vi "main.vi"() -> ()   [LabVIEW 2016]
panel:
  out "Y":dbl(slide) scale=0.0..720.0
  out "X":dbl(slide) scale=0.0..1280.0
  out "Ball Y Position":dbl
  out "Ball X Position":dbl
  out "Frame Rate":dbl
  in  "Stop (F)":bool
  out "Image Out":T1(plugin-control)
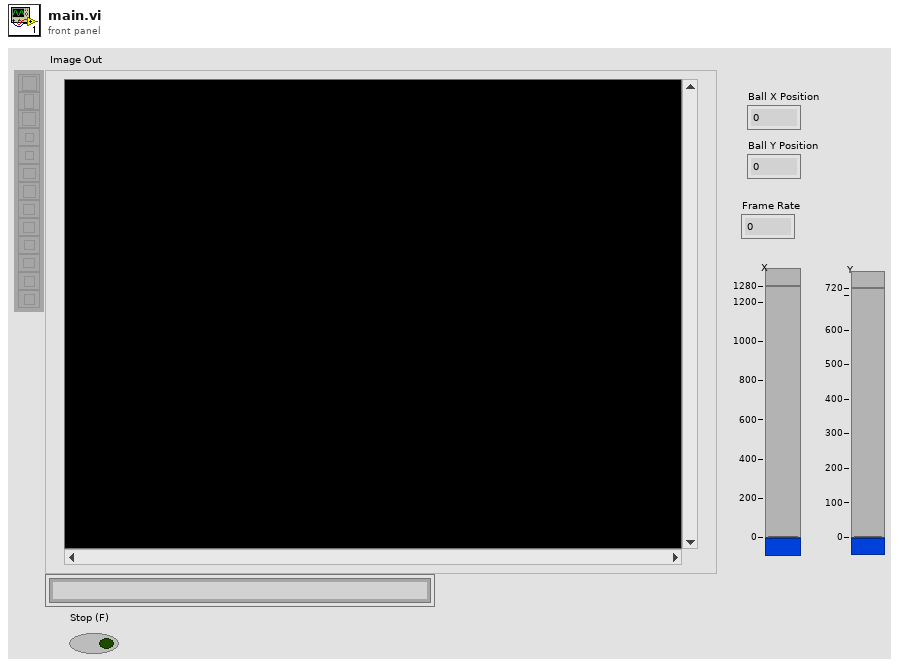
[diagram p1: front panel]
types:
  T1 = typedef "IMAQ Image.ctl" = refnum<image>
  T2 = cluster{"Label":string, "Score":i32, "Angle":dbl, "Location":cluster{"X":dbl, "Y":dbl}, "Bounding Box":cluster{"X":dbl, "Y":dbl}[], "Object Found?":bool}[]
  T3 = cluster{"Label":string, "Score":i32, "Angle":dbl, "Location":cluster{"X":dbl, "Y":dbl}, "Bounding Box":cluster{"X":dbl, "Y":dbl}[], "Object Found?":bool}
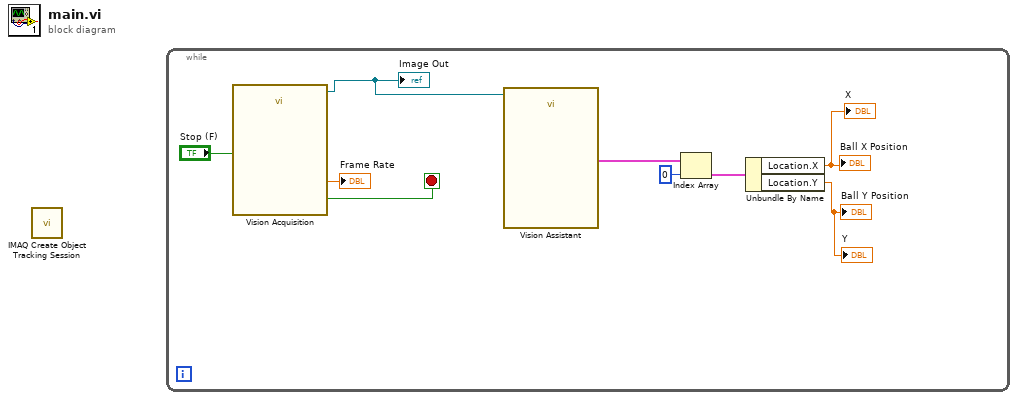
[diagram p0: block diagram]
diagram:
  n1 = call "IMAQ Create Object Tracking Session"() -> ()  [unwired: 10 in, 2 out]
  n2 = while {
    stop <- w8 stop-if-true
    n3 = call "Vision Acquisition"("Stop (F)"="Stop (F)") -> ("Image Out"=w6:T1, "Frame Rate"=→"Frame Rate":dbl, "Stopped"=w8:bool)  [unwired: 23 in, 1 out]
    "Image Out" <- w6
    n4 = call "Vision Assistant"("Image In"=w6) -> ("Objects (pixel) (Object Tracking 1)"=w5:T2)  [unwired: 22 in, 4 out]
    n5 = Index Array(array=w5, index=0) -> (element=w3:T3)
    n6 = Unbundle By Name(w3) -> ("Location.X"=→"Ball X Position" →"X":dbl, "Location.Y"=→"Ball Y Position" →"Y":dbl)
  }
